vi "Destroy command queue.vi"(8 "error in (no error)":errorcluster) -> (0 "error out":errorcluster)   [LabVIEW 2020, in "queue_display_loop_1.lvlib"]
uses:
  queue_display_loop_1.lvlib
panel:
  # "Development\ncontrols/indicators useful for development and testing, but which are not outputs of the VI"
  # "Input\nInputs to the VI"
  # "Output\nOutputs of the VI"
  # "Description\n\nBlank VI with error handling case. \n\nSummarize the use of this VI in this space."
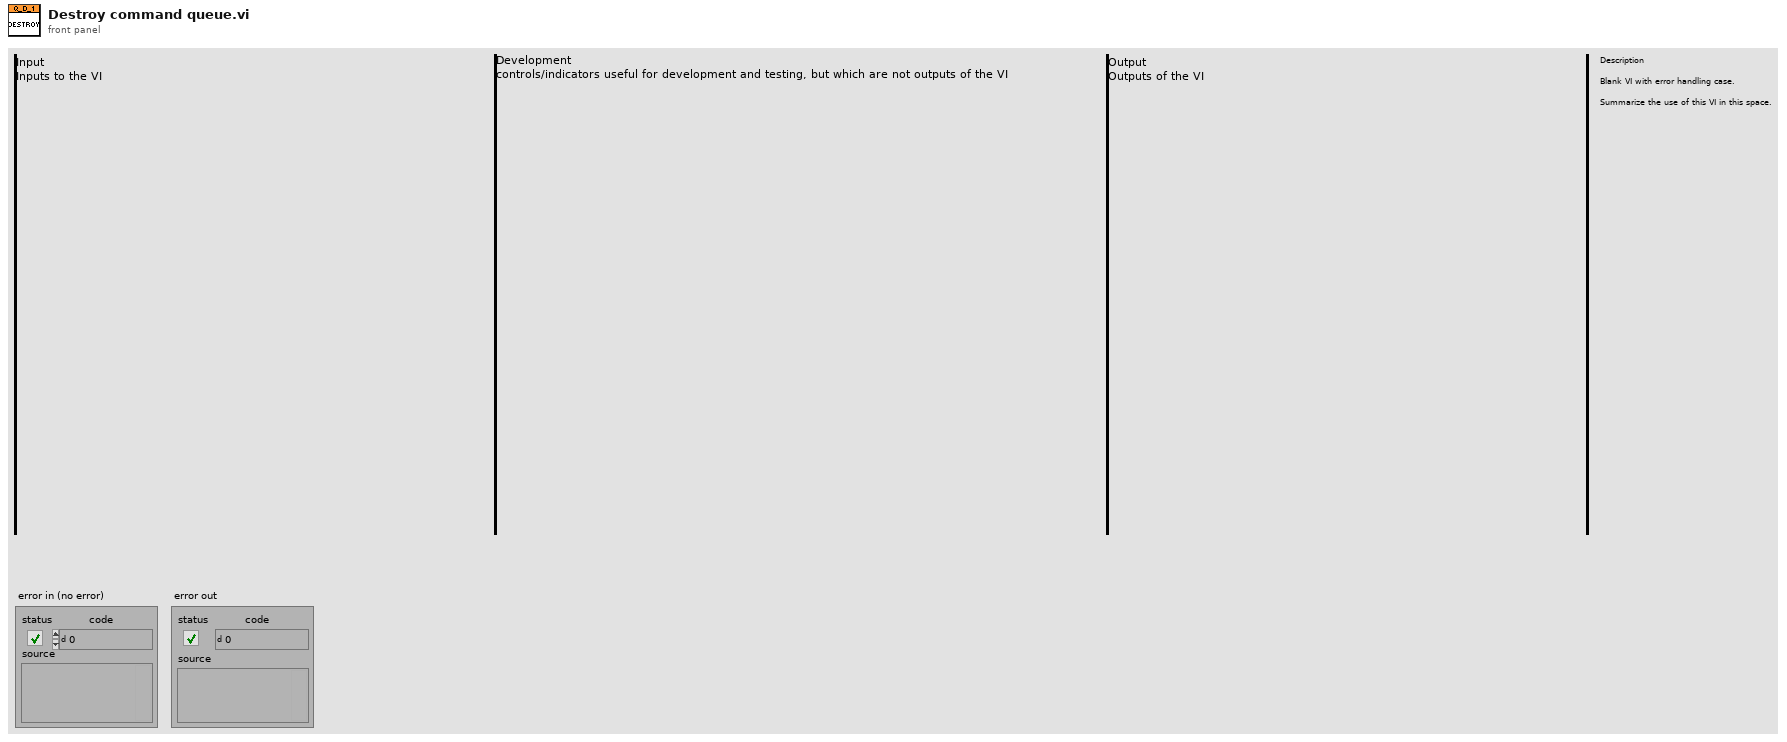
[diagram p1: front panel]
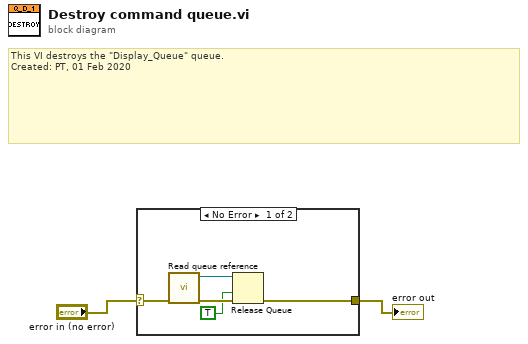
[diagram p0: block diagram]
diagram:
  # "This VI destroys the \"Display_Queue\" queue.\nCreated: PT, 01 Feb 2020"
  n1 = case shown="No Error" "error in (no error)" {
    selector: "error in (no error)" -> [w7 w8]
    tunnel: [w6 w8] -> w1
    frame No Error {
      n2 = call "Read queue reference.vi"("error in (no error)"=w7) -> ("error out"=w5:errorcluster, "ALA_Display_Queue ref"=w4:refnum<queue>)  [unwired: 9 in]
      n3 = Release Queue(queue=w4, force destroy? (F)=TRUE, error in (no error)=w5) -> (error out=w6:errorcluster)  [unwired: 2 out]
    }
    frame Error {
    }
  }
  "error out" <- w1
